vi "Write Actual Value (Single).vi"(8 "error in":errorcluster, 9 "Channel Index":i32=1, 10 "Actual Value":dbl, 11 "Actual Value in":refnum<class "Actual Value.lvclass">) -> (0 "error out":errorcluster, 3 "Actual Value out":refnum<class "Actual Value.lvclass">)   [LabVIEW 2023, in "Actual Value.lvclass"]
uses:
  Actual Value.lvclass
  Actual Value.lvclass/Actual Value.ctl
  <vilib>/ADAS Replay HIL/Channels/Tag Wrapper/Polymorphic/Write Channel (Double).vi
  <vilib>/ADAS Replay HIL/Channels/Tag Wrapper/Polymorphic/Write Channel (Double).vi/cccb8e89-591f-4bb4-9d4e-ae06ba1f5498.vi
  <vilib>/ADAS Replay HIL/Channels/Tag Wrapper/Polymorphic/Write Channel (Double).vi/cccb8e89-591f-4bb4-9d4e-ae06ba1f5498.vi/4bc1c15b-36ab-481f-b8dd-c64075ce723a.vi
  <vilib>/ADAS Replay HIL/Channels/Tag Wrapper/Polymorphic/Write Channel (Double).vi/cccb8e89-591f-4bb4-9d4e-ae06ba1f5498.vi/d83cb72b-7713-41fc-a3d1-682de79cf574.vi
  <vilib>/ADAS Replay HIL/Channels/Tag Wrapper/Tag Wrapper.lvlib
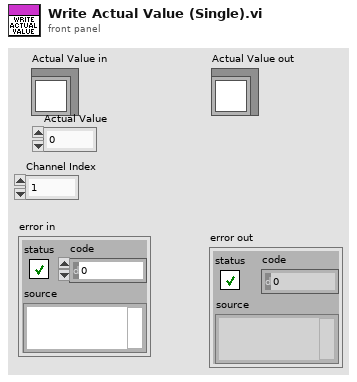
[diagram p1: front panel]
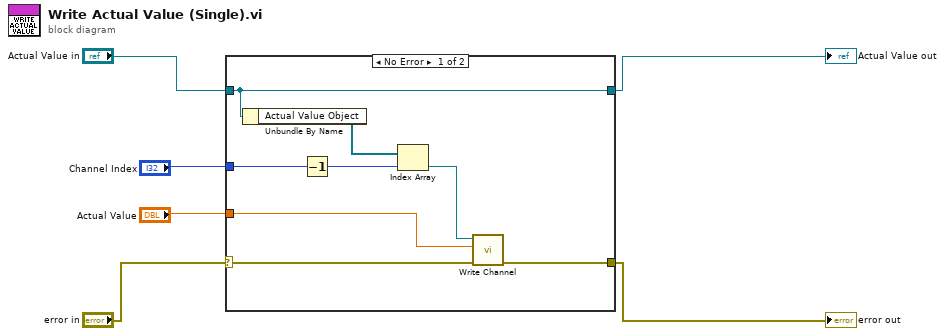
[diagram p0: block diagram]
diagram:
  n1 = case shown="No Error" "error in" {
    selector: "error in" -> [w14 w15]
    tunnel: [w13 w15] -> w3
    tunnel: [w11 w16] -> w5
    tunnel: "Actual Value in" -> [w11 w16]
    tunnel: "Actual Value" -> [w12 _]
    tunnel: "Channel Index" -> [w8 _]
    frame No Error {
      n2 = Unbundle By Name(w11) -> ("Actual Value Object"=w10:refnum<k21>[])
      n3 = Decrement(x=w8) -> (x-1=w7:i32)
      n4 = Index Array(array=w10, index=w7) -> (element=w9:refnum<k21>)
      n5 = call-poly <vilib>:"Write Channel.vi"("error in"=w14, "Value to Write"=w12, "ADAS HIL Channel in"=w9) -> ("error out"=w13:errorcluster)  [unwired: 6 in, 2 out]
    }
    frame Error {
    }
  }
  "error out" <- w3
  "Actual Value out" <- w5
